vi "Read AO.Channels.vi"(8 "error in (no error)":errorcluster, 11 "DAQ in":refnum<class "DAQ.lvclass">) -> (0 "error out":errorcluster, 2 "AO.Channels":T1, 3 "DAQ out":refnum<class "DAQ.lvclass">)   [LabVIEW 2016]
uses:
  DAQ.lvclass
  C:/Program Files (x86)/National Instruments/LabVIEW 2016/vi.lib/JKI/JKI SMO/SMO/SMO.lvclass
  Typedefs/PrivateEvents--DAQ.AO.Channels.ctl
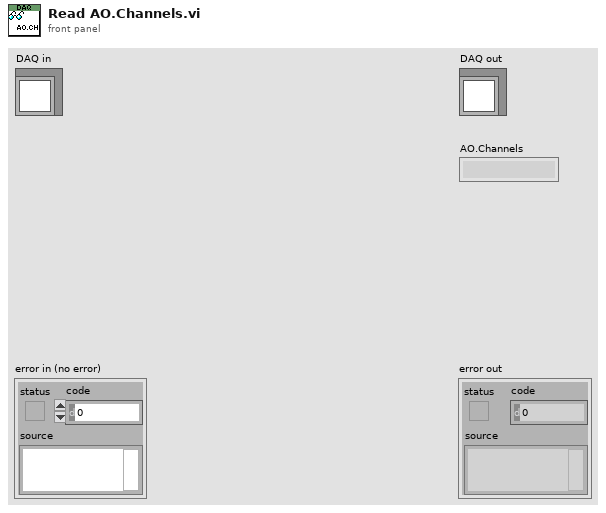
[diagram p1: front panel]
types:
  T1 = typedef "PrivateEvents--DAQ.AO.Channels.ctl" = string
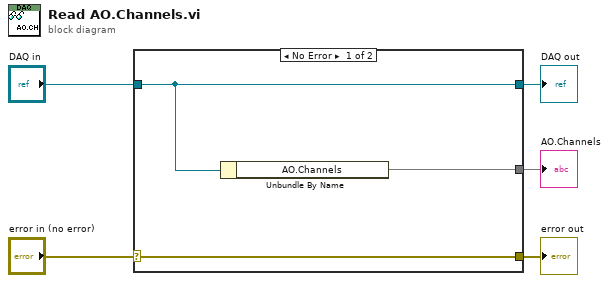
[diagram p0: block diagram]
diagram:
  n1 = case shown="No Error" "error in (no error)" {
    selector: "error in (no error)" -> [w8 w9]
    tunnel: [w8 w9] -> w4
    tunnel: [w7 w10] -> w2
    tunnel: "DAQ in" -> [w7 w10]
    tunnel: [w6 _] -> w1
    frame No Error {
      n2 = Unbundle By Name(w7) -> ("AO.Channels"=w6)
    }
    frame Error {
    }
  }
  "error out" <- w4
  "DAQ out" <- w2
  "AO.Channels" <- w1
